vi "MQTT_Simple_Connect_and_Subscribe.vi"() -> ()   [LabVIEW 2015, in "MQTT_Functions.lvlib"]
uses:
  MQTT_Functions.lvlib
  Controls/Connect_Flags.ctl
  Controls/QoS.ctl
  Controls/Connection_Return_Codes.ctl
  Controls/MessageType.ctl
  Controls/DUP_Flag.ctl
  Controls/Retain_Flag.ctl
  Controls/User_Info.ctl
panel:
  out "Messages":T2(array[cluster])
  in  "Stop Reading":bool
  in  "MQTT Broker":cluster{"address (IP)":string, "port":u16}={"address (IP)"="broker.mqttdashboard.cobroker.mqttdashboard.com", "port"=1883}
  in  "Subscription Info Array":cluster{"Topic":string, "QoS":T3}[](array[cluster])=[{"Topic"="dcsquare/cubes/1/light", "QoS"=enum."At least once"}]
  out "Granted QoS Levels":T3[](array[typedef])
  out "Connection Status":T4=enum."Connection refused: Server unavailable"
  in  "Connect Flags":T5
  in  "Client ID":string="NodeE-12345"
  out "error out":errorcluster
  in  "error in (no error)":errorcluster
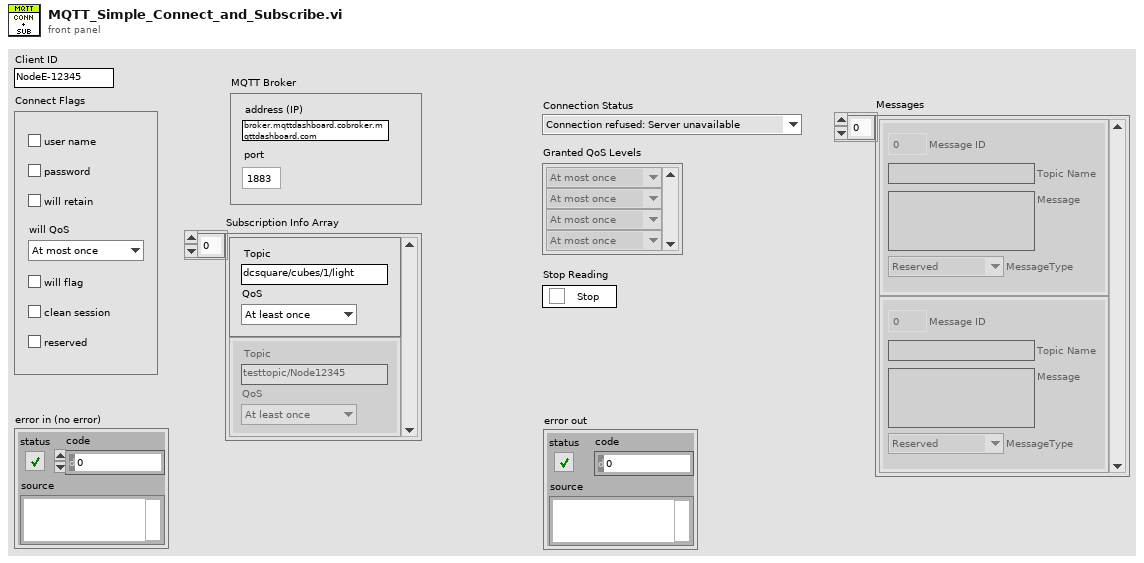
[diagram p1: front panel]
types:
  T1 = typedef "MQTT_Functions.lvlib/MessageType.ctl" = enum32{"Reserved", "CONNECT", "CONNACK", "PUBLISH", "PUBACK", "PUBREC", "PUBREL", "PUBCOMP", "SUBSCRIBE", "SUBACK", "UNSUBSCRIBE", "UNSUBACK", "PINGREQ", "PINGRESP", "DISCONNECT", "Reserved2"}
  T2 = cluster{"Message ID":u16, "Topic Name":string, "Message ":string, "MessageType":T1}[]
  T3 = typedef "MQTT_Functions.lvlib/QoS.ctl" = enum8{"At most once", "At least once", "Exactly once", "Reserved"}
  T4 = typedef "MQTT_Functions.lvlib/Connection_Return_Codes.ctl" = enum16{"Connection accepted", "Connection refused: unacceptable protocol version", "Connection refused: identifier rejected", "Connection refused: Server unavailable", "Connection refused: bad user name or password", "Connection refused: not authorized"}
  T5 = typedef "MQTT_Functions.lvlib/Connect_Flags.ctl" = cluster{"user name":bool, "password":bool, "will retain":bool, "will flag":bool, "clean session":bool, "reserved":bool, "will QoS":T3}
  T6 = typedef "MQTT_Functions.lvlib/User_Info.ctl" = cluster{"User Name":string, "Password":string}
  T7 = cluster{"Message ID":u16, "Topic Name":string, "Message":string, "MessageType":T1}[]
  T8 = typedef "MQTT_Functions.lvlib/DUP_Flag.ctl" = bool
  T9 = typedef "MQTT_Functions.lvlib/Retain_Flag.ctl" = bool
  T10 = cluster{"QoS":T3, "DUP":T8, "Retain":T9, "Keep Alive (sec)":u16}
  T11 = cluster{"Message ID":u16, "Topic Name":string, "Message":string, "MessageType":T1}
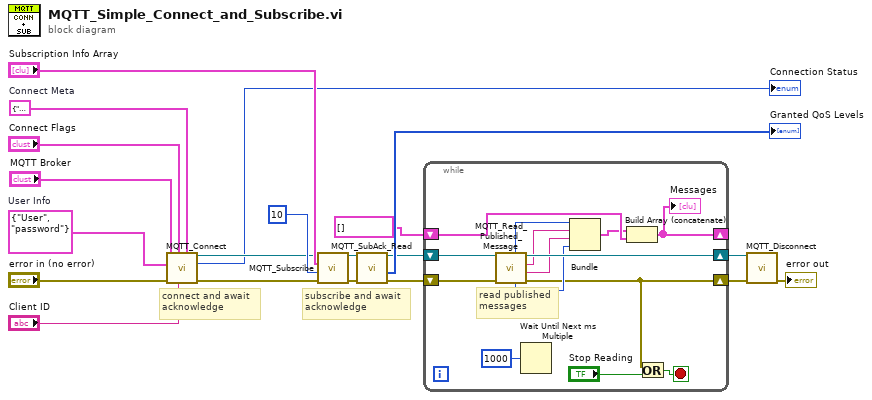
[diagram p0: block diagram]
diagram:
  w1 = T6 {"User Name"="User", "Password"="password"}  # User Info
  w17 = T10 {"QoS"=enum."At least once", "DUP"=FALSE, "Retain"=FALSE, "Keep Alive (sec)"=10}  # Connect Meta
  # "connect and await\nacknowledge"
  # "subscribe and await\nacknowledge"
  n1 = call "MQTT_Connect.vi"("Connect Meta"=w17, "Client ID"="Client ID", "Connect Flags"="Connect Flags", "error in (no error)"="error in (no error)", "User Info"=w1, "MQTT Broker"="MQTT Broker") -> ("error out"=w2:errorcluster, "Connection Status"=→"Connection Status":T4, "connection ID out"=w4:refnum<k5>)  [unwired: 3 in]
  n2 = call "MQTT_Subscribe.vi"("error in (no error)"=w2, "Message ID"=u16 10, "Subscription Info Array"="Subscription Info Array", "connection ID"=w4) -> ("error out"=w13:errorcluster, "connection ID out"=w14:refnum<k5>)  [unwired: 6 in]
  n3 = call "MQTT_SubAck_Read.vi"("error in (no error)"=w13, "connection ID"=w14) -> ("error out"=w11:errorcluster, "Granted QoS Levels"=→"Granted QoS Levels":T3[], "connection ID out"=w10:refnum<k5>)  [unwired: 7 in]
  n4 = while {
    shift-right: [w23] -> _
    shift-left: T7 [] ("Array") -> [w22]
    shift-right: [w24] -> w8
    shift-left: w11 -> [w34]
    shift-right: [w32] -> w9
    shift-left: w10 -> [w33]
    stop <- w26 stop-if-true
    # "read published\nmessages"
    n5 = call "MQTT_Read_Published_Message.vi"("error in (no error)"=w34, "connection ID"=w33) -> ("error out"=w24:errorcluster, "Message"=w29:string, "Topic Name"=w30:string, "connection ID out"=w32:refnum<k5>, "MessageType"=w28:T1, "Message ID"=w31:u16)  [unwired: 4 in]
    n6 = Wait Until Next ms Multiple(millisecond multiple=u32 1000) -> ()  [unwired: 1 out]
    n7 = Bundle("Message ID"=w31, "Topic Name"=w30, "Message"=w29, "MessageType"=w28) -> (w21:T11)  [unwired: 1 in]
    n8 = Build Array (concatenate)(w21, w22) -> (w23:T7)
    "Messages" <- w23
    n9 = Or(x=w24, y="Stop Reading") -> (x .or. y?=w26:bool)
  }
  n10 = call "MQTT_Disconnect.vi"("error in (no error)"=w8, "connection ID"=w9) -> ("error out"=→"error out":errorcluster)  [unwired: 9 in]
